vi "Initialize and Sort Key Values.vi"() -> (8 "refnum":T1, 11 "Preferences":string[][](array[string]))   [LabVIEW 2015]
uses:
  <vilib>/Utility/config.llb/Config Data RefNum.ctl
  <vilib>/Utility/config.llb/Read Key (String).vi
  <vilib>/Utility/config.llb/NI_LVConfig.lvlib
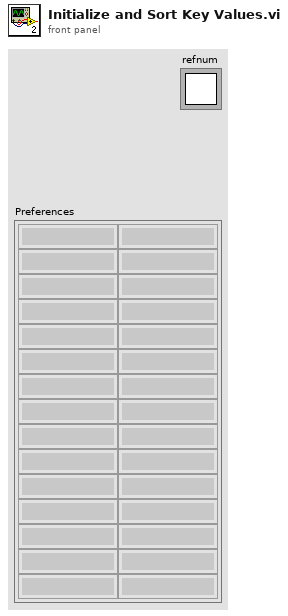
[diagram p1: front panel]
types:
  T1 = typedef "NI_LVConfig.lvlib/Config Data RefNum.ctl" = refnum<k1>
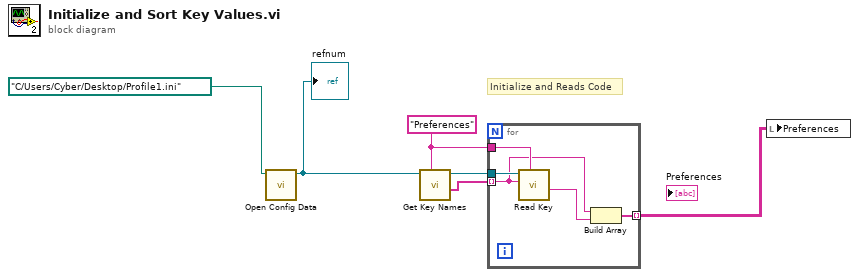
[diagram p0: block diagram]
diagram:
  w5 = "Preferences" ("section")
  # "Initialize and Reads Code"
  n1 = call <vilib>:"Open Config Data.vi"("configuration file path"=path "C:/Users/Cyber/Desktop/Profile1.ini" ("path")) -> ("refnum"=w1:T1)  [unwired: 8 in, 2 out]
  "refnum" <- w1
  n2 = call <vilib>:"Get Key Names.vi"("section"=w5, "refnum"=w1) -> ("key names"=w6:string[], "refnum out"=w4:T1)  [unwired: 6 in, 2 out]
  n3 = for {
    tunnel: w6 -> [w9] mode=indexing
    tunnel: w4 -> [w11]
    tunnel: w5 -> [w10]
    tunnel: [w7] -> w3 mode=indexing
    n4 = call-poly <vilib>:"Read Key.vi"("section"=w10, "key"=w9, "refnum"=w11) -> ("value"=w8:string)  [unwired: 5 in, 3 out]
    n5 = Build Array(w9, w8) -> (w7:string[])
  }
  n6 = local write "Preferences"(w3) -> ()
